vi "Acquisition Message Loop.vi"(8 "error in (no error)":errorcluster, 9 "Data Queue":refnum<queue>, 10 "Data Notifier":refnum<notifier>, 11 "Message Queues":T3) -> (0 "error out":errorcluster)   [LabVIEW 2020, in "Acquisition.lvlib"]
doc: "Message loop for handling messages pertaining to the acquisition of data from the hardware."
uses:
  Acquisition.lvlib
  MESSAGE_QUEUE/All Message Queues.ctl
  MESSAGE_QUEUE/Message Cluster.ctl
  SETTING/data_Queue.ctl
  SETTING/data_Display.ctl
  SETTING/clustOA.ctl
  <vilib>/Analysis/Matrix/Datatypes/RealMatrix.ctl
  HardwareConfiguration.ctl
  CLASS/Image Acquisition Class/Camera.lvclass
  MIRROR/mirror.lvclass
  MIRROR/SIMU_MIRROR/SIMU_MIRROR.lvclass
  D:/USERS/MONTRI/BABYDOL/LABVIEW/EXEMPLE_ARCHITECTURE/acquImageCont_Sav2FITS/MIRROR/mirror.lvclass
  MESSAGE_QUEUE/Message Queue.lvlib
  <vilib>/Analysis/Matrix/NI_Matrix.lvlib
panel:
  out "Cluster 3":cluster{"processedFPS":dbl, "Buffer Number":u32}
  in  "clustPointagFin":T1
  out "File Path Control":path
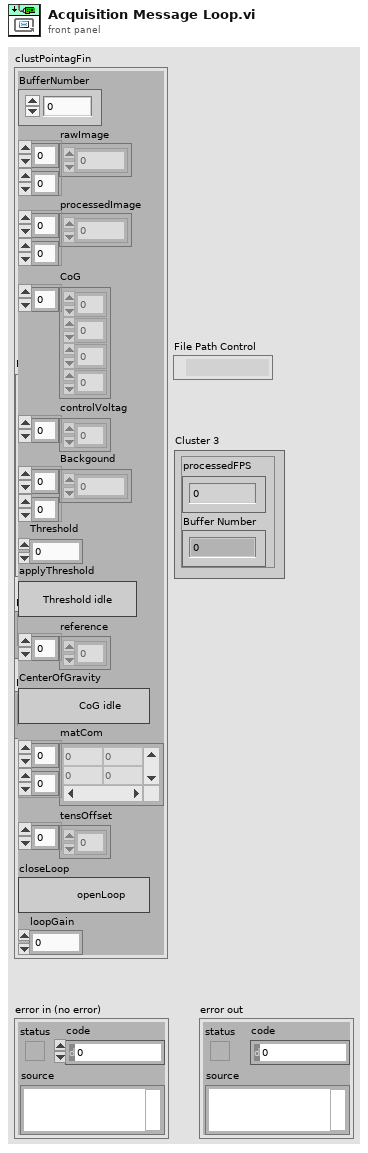
[diagram p1: front panel]
types:
  T1 = typedef "clustOA.ctl" = cluster{"BufferNumber":u32, "rawImage":u16[][], "processedImage":sgl[][], "CoG":dbl[], "controlVoltag":dbl[], "Backgound":sgl[][], "Threshold":dbl, "applyThreshold":bool, "reference":dbl[], "CenterOfGravity":bool, "matCom":T2, "tensOffset":dbl[], "closeLoop":bool, "loopGain":dbl}
  T2 = typedef "NI_Matrix.lvlib/RealMatrix.ctl" = dbl[][]
  T3 = typedef "Message Queue.lvlib/All Message Queues.ctl" = cluster{"UI":refnum<queue>, "Acquisition":refnum<queue>, "Logging":refnum<queue>}
  T4 = typedef "Acquisition.lvlib/HardwareConfiguration.ctl" = cluster{"Camera.lvclass":refnum<class "Camera.lvclass">, "InClusTiming 2":cluster{"Pixelclock":i32, "Exposure":dbl, "ExposureTimeBase":u16, "Framerate":dbl, "TriggerMode":u16}, "ROI":cluster{"PosX":i32, "PosY":i32, "Width":i32, "Height":i32}, "File Path Control":path, "mirror.lvclass":refnum<class "mirror.lvclass">}
  T5 = cluster{"threshold":bool, "thresholdValue (0)":dbl}
  T6 = cluster{"Pixelclock":i32, "Exposure":dbl, "ExposureTimeBase":u16, "Framerate":dbl, "TriggerMode":u16}
  T7 = cluster{"PosX":i32, "PosY":i32, "Width":i32, "Height":i32}
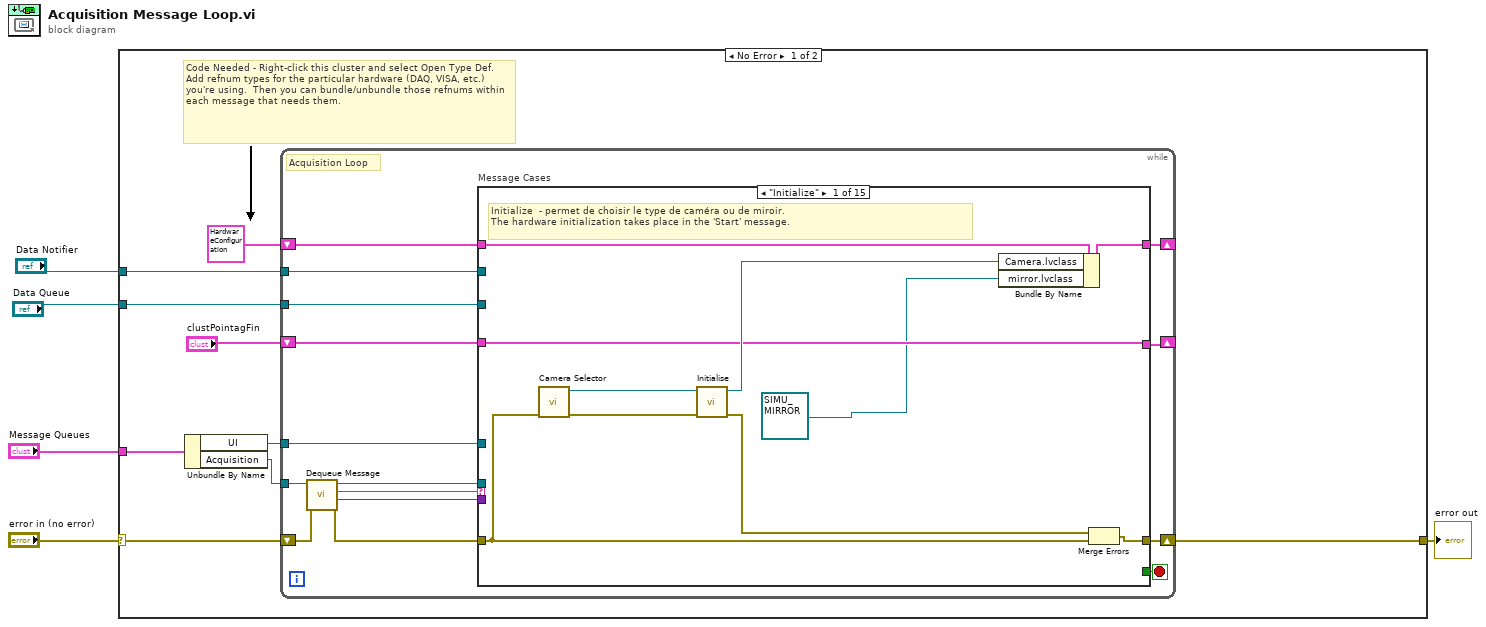
[diagram p0: block diagram]
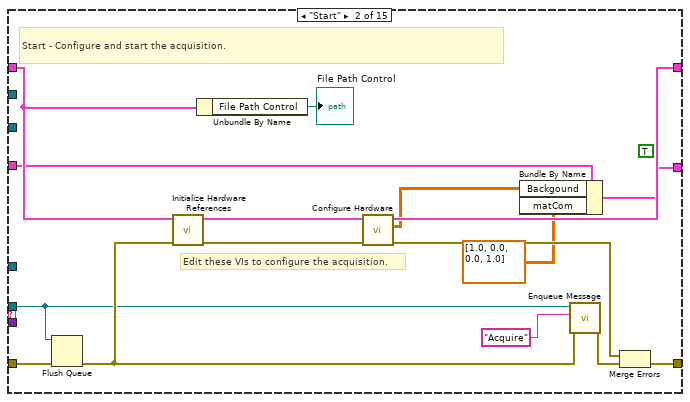
[diagram p2: hidden frame]
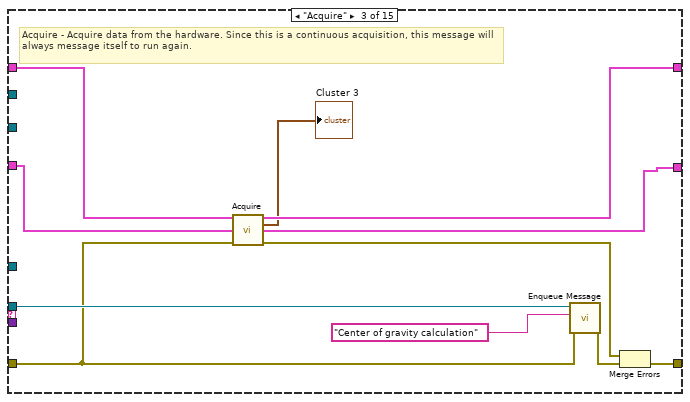
[diagram p3: hidden frame]
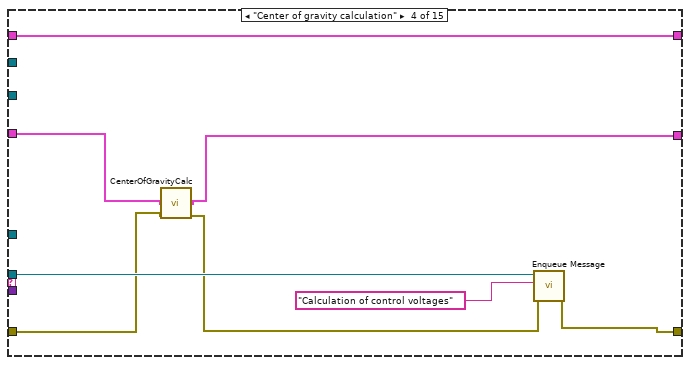
[diagram p4: hidden frame]
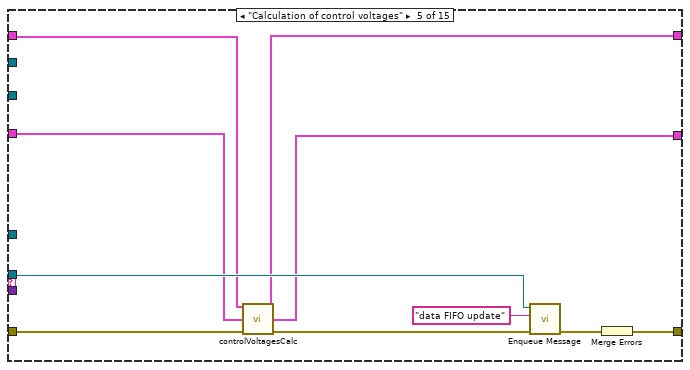
[diagram p5: hidden frame]
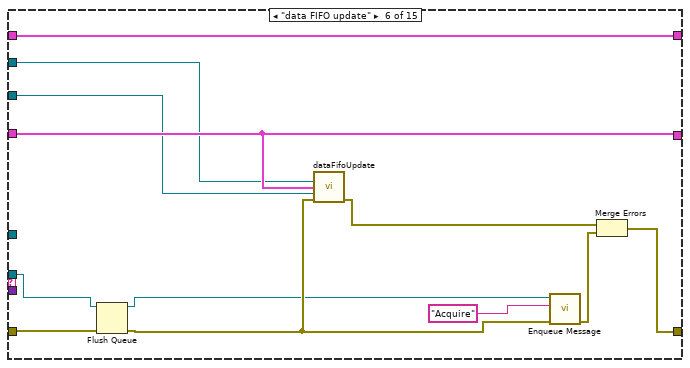
[diagram p6: hidden frame]
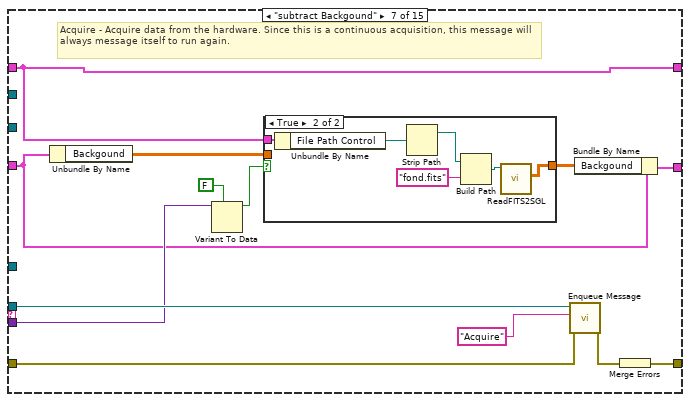
[diagram p7: hidden frame]
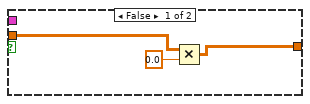
[diagram p8: hidden frame]
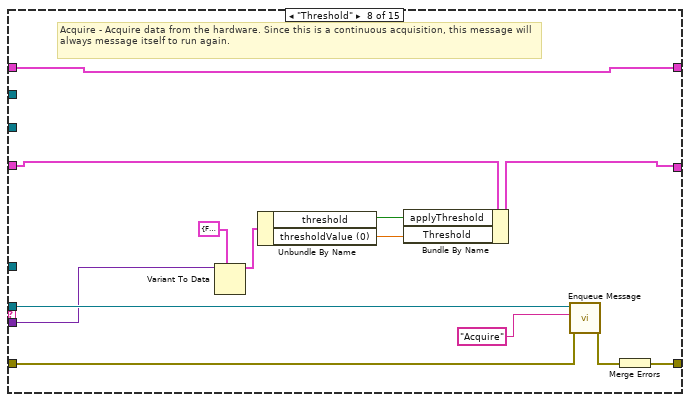
[diagram p9: hidden frame]
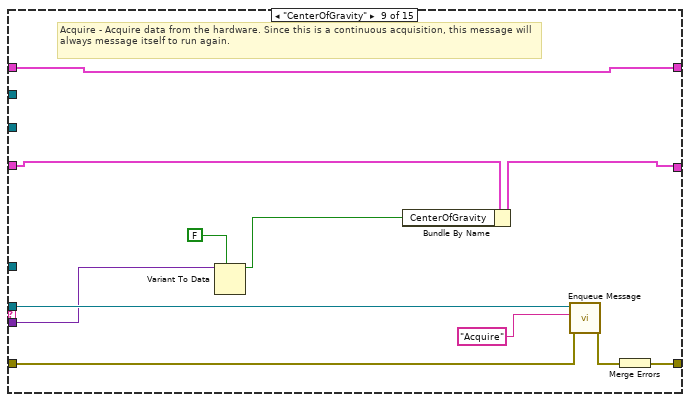
[diagram p10: hidden frame]
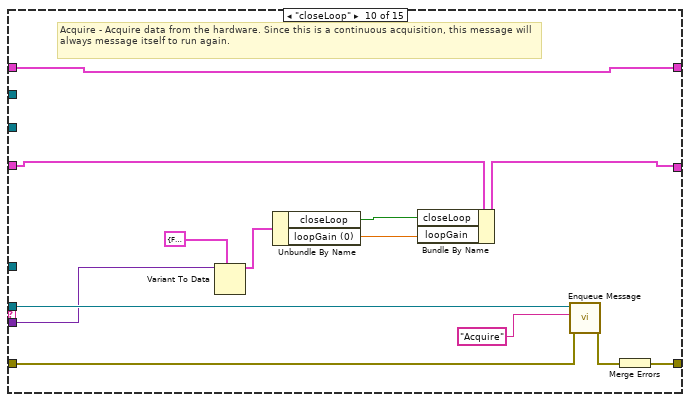
[diagram p11: hidden frame]
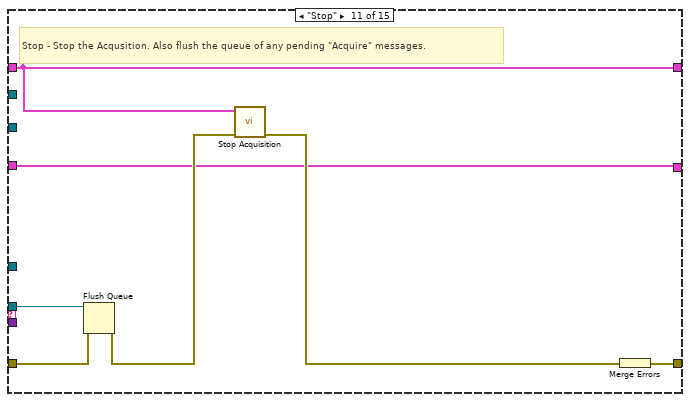
[diagram p12: hidden frame]
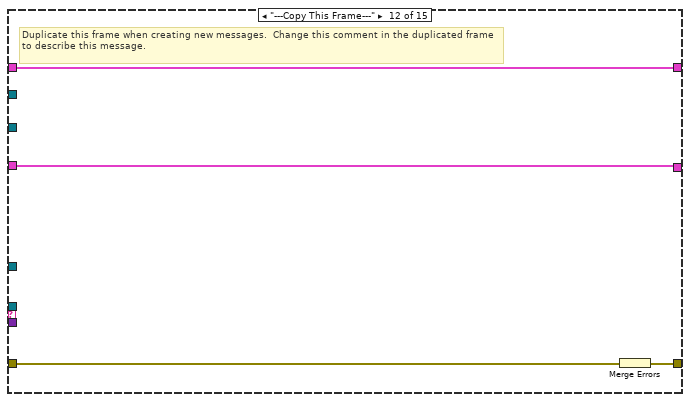
[diagram p13: hidden frame]
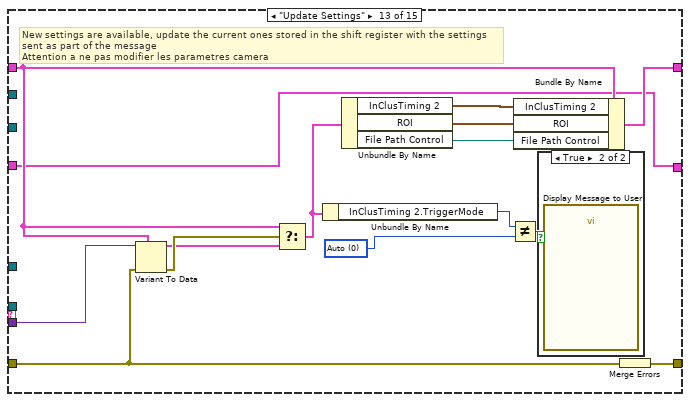
[diagram p14: hidden frame]
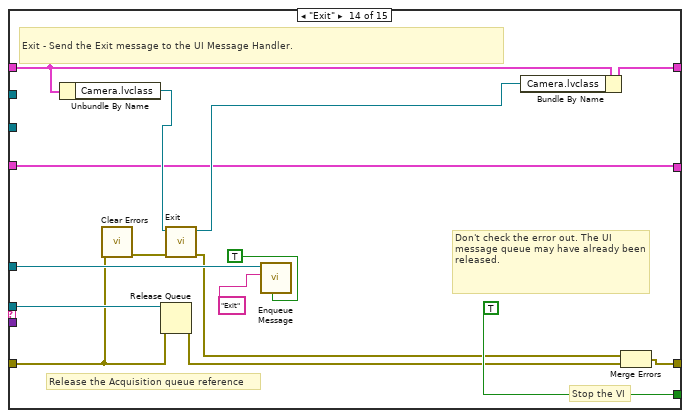
[diagram p16: hidden frame]
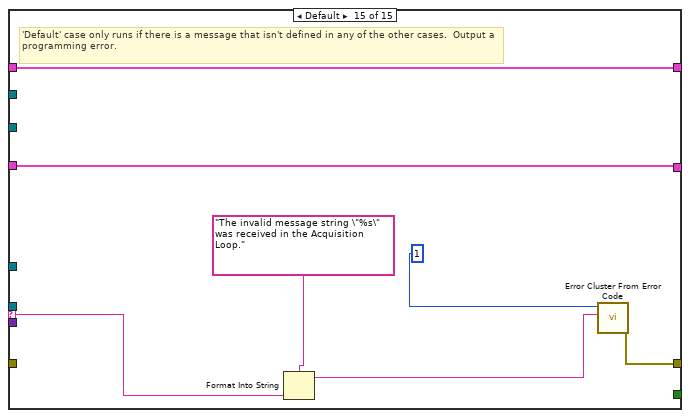
[diagram p17: hidden frame]
diagram:
  n1 = case shown="No Error" "error in (no error)" {
    selector: "error in (no error)" -> [w11 w204]
    tunnel: "Message Queues" -> [w14 _]
    tunnel: [w12 w204] -> w4
    tunnel: "Data Notifier" -> [w9 _]
    tunnel: "Data Queue" -> [w8 _]
    frame No Error {
      # "Code Needed - Right-click this cluster and select Open Type Def.  Add refnum types for the particular hardware (DAQ, VISA, etc.) you're using.  Then you can bundle/unbundle those refnums within each message that needs them."
      n2 = Unbundle By Name(w14) -> ("UI"=w10:refnum<queue>, "Acquisition"=w13:refnum<queue>)
      n3 = while {
        tunnel: w13 -> [w22]
        shift-right: [w28] -> _
        shift-left: T4 {"Camera.lvclass"=refnum, "InClusTiming 2"={"Pixelclock"=0, "Exposure"=0.0, "ExposureTimeBase"=0, "Framerate"=0.0, "TriggerMode"=0}, "ROI"={"PosX"=0, "PosY"=0, "Width"=0, "Height"=0}, "File Path Control"=path "", "mirror.lvclass"=refnum} -> [w29]
        shift-right: [w26] -> w12
        shift-left: w11 -> [w25]
        tunnel: w10 -> [w21]
        tunnel: w9 -> [w20]
        tunnel: w8 -> [w19]
        shift-right: [w15] -> _
        shift-left: "clustPointagFin" -> [w18]
        stop <- w27 stop-if-true
        # "Acquisition Loop"
        n4 = call "Dequeue Message.vi"("error in (no error)"=w25, "Message Queue"=w22) -> ("error out"=w24:errorcluster, "Message Data"=w17:variant, "Message"=w16:string, "dup Message Queue"=w23:refnum<queue>)  [unwired: 6 in]
        n5 = case "Message Cases" shown="\"Initialize\"" w16 {
          selector: w16 -> [_ _ _ _ _ _ _ _ _ _ _ _ _ _ w201]
          tunnel: w23 -> [_ w40 w64 w71 w83 w86 w107 w129 w140 w153 w158 _ _ w190 _]
          tunnel: w24 -> [w32 w42 w63 w68 w80 w88 w106 w128 w139 w152 w161 w166 w177 w189 _]
          tunnel: [w39 w55 w66 w72 w78 w89 w109 w131 w142 w155 w162 w164 w181 w195 w199] -> w26
          tunnel: w29 -> [w38 w48 w59 w74 w77 w95 w104 w126 w137 w150 w157 w165 w176 w186 w203]
          tunnel: [w36 w49 w61 w74 w76 w95 w104 w126 w137 w150 w157 w165 w175 w184 w203] -> w28
          tunnel: [_ _ _ _ _ _ _ _ _ _ _ _ _ TRUE _] -> w27
          tunnel: w17 -> [_ _ _ _ _ _ w103 w125 w136 w149 _ _ w180 _ _]
          tunnel: w21 -> [_ _ _ _ _ _ _ _ _ _ _ _ _ w194 _]
          tunnel: w20 -> [_ _ _ _ _ w92 _ _ _ _ _ _ _ _ _]
          tunnel: w19 -> [_ _ _ _ _ w93 _ _ _ _ _ _ _ _ _]
          tunnel: w18 -> [w31 w46 w58 w70 w82 w94 w100 w124 w135 w148 w156 w163 w167 w182 w197]
          tunnel: [w31 w45 w57 w69 w75 w94 w98 w123 w134 w147 w156 w163 w167 w182 w197] -> w15
          frame "Initialize" {
            # "Initialize  - permet de choisir le type de caméra ou de miroir. \nThe hardware initialization takes place in the 'Start' message."
            n6 = call "Camera Selector.vi"("error in (no error)"=w32) -> ("error out"=w34:errorcluster, "Image Acquisition out"=w33:refnum<class "Camera.lvclass">)  [unwired: 9 in]
            n7 = call-dynamic "Initialise.vi"("error in (no error)"=w34, "Image Acquisition in"=w33) -> ("error out"=w37:errorcluster, "Image Acquisition out"=w35:refnum<class "Camera.lvclass">)  [unwired: 8 in]
            n8 = Bundle By Name(cluster=w38, "Camera.lvclass"=w35, "mirror.lvclass"=refnum<class "SIMU_MIRROR.lvclass"> refnum ("SIMU_MIRROR.lvclass")) -> (w36:T4)
            n9 = Merge Errors(w37, w32) -> (w39:errorcluster)
          }
          frame "Start" {
            (unwired) TRUE ("bUseBuffer0")
            # "Edit these VIs to configure the acquisition."
            # "Start - Configure and start the acquisition."
            n10 = Flush Queue(queue=w40, error in (no error)=w42) -> (error out=w41:errorcluster)  [unwired: 2 out]
            n11 = call "Initialize Hardware References.vi"("error in (no error)"=w41, "Cluster"=w48) -> ("error out"=w53:errorcluster, "Cluster 2"=w50:T4)  [unwired: 8 in]
            n12 = Unbundle By Name(w48) -> ("File Path Control"=→"File Path Control":path)
            n13 = call "Configure Hardware.vi"("error in (no error)"=w53, "Cluster"=w50) -> ("error out"=w52:errorcluster, "initialized array"=w44:sgl[][], "Cluster 2"=w49:T4)  [unwired: 7 in]
            n14 = Bundle By Name(cluster=w46, "Backgound"=w44, "matCom"=T2 [[1.0, 0.0], [0.0, 1.0]]) -> (w45:T1)
            n15 = call "Enqueue Message.vi"("error in (no error)"=w41, "Message"="Acquire", "Message Queue"=w40) -> ("error out"=w54:errorcluster)  [unwired: 7 in, 1 out]
            n16 = Merge Errors(w52, w54) -> (w55:errorcluster)
          }
          frame "Acquire" {
            # "Acquire - Acquire data from the hardware. Since this is a continuous acquisition, this message will always message itself to run again."
            n17 = call "Acquire.vi"("Cluster"=w59, "clustPointagFin"=w58, "error in (no error)"=w63) -> ("Cluster 2"=w61:T4, "clustBufferNumber"=→"Cluster 3":cluster{"processedFPS":dbl, "Buffer Number":u32}, "clustPointagFin"=w57:T1, "error out"=w62:errorcluster)  [unwired: 9 in]
            n18 = call "Enqueue Message.vi"("error in (no error)"=w63, "Message"="Center of gravity calculation", "Message Queue"=w64) -> ("error out"=w65:errorcluster)  [unwired: 7 in, 1 out]
            n19 = Merge Errors(w62, w65) -> (w66:errorcluster)
          }
          frame "Center of gravity calculation" {
            n20 = call "CenterOfGravityCalc.vi"("clustPointagFin"=w70, "error in (no error)"=w68) -> ("clustPointagFin"=w69:T1, "error out"=w67:errorcluster)  [unwired: 12 in]
            n21 = call "Enqueue Message.vi"("error in (no error)"=w67, "Message"="Calculation of control voltages", "Message Queue"=w71) -> ("error out"=w72:errorcluster)  [unwired: 7 in, 1 out]
          }
          frame "Calculation of control voltages" {
            n22 = call "controlVoltagesCalc.vi"("Camera"=w77, "clustPointagFin"=w82, "error in (no error)"=w80) -> ("output cluster"=w76:T4, "clustPointagFin"=w75:T1, "error out"=w81:errorcluster)  [unwired: 10 in]
            n23 = call "Enqueue Message.vi"("error in (no error)"=w81, "Message"="data FIFO update", "Message Queue"=w83) -> ("error out"=w79:errorcluster)  [unwired: 7 in, 1 out]
            n24 = Merge Errors(w79) -> (w78:errorcluster)
          }
          frame "data FIFO update" {
            n25 = Flush Queue(queue=w86, error in (no error)=w88) -> (queue out=w85:refnum<queue>, error out=w87:errorcluster)  [unwired: 1 out]
            n26 = call "dataFifoUpdate.vi"("Data Notifier"=w92, "clustPointagFin"=w94, "Data Queue"=w93, "error in (no error)"=w87) -> ("error out"=w91:errorcluster)  [unwired: 11 in]
            n27 = call "Enqueue Message.vi"("error in (no error)"=w87, "Message"="Acquire", "Message Queue"=w85) -> ("error out"=w90:errorcluster)  [unwired: 7 in, 1 out]
            n28 = Merge Errors(w91, w90) -> (w89:errorcluster)
          }
          frame "subtract Backgound" {
            # "Acquire - Acquire data from the hardware. Since this is a continuous acquisition, this message will always message itself to run again."
            n29 = Unbundle By Name(w100) -> ("Backgound"=w99:sgl[][])
            n30 = Variant To Data(type=FALSE, Variant=w103) -> (data=w101:bool)  [unwired: 1 in, 1 out]
            n31 = case shown="True" w101 {
              tunnel: w104 -> [_ w118]
              tunnel: [w111 w117] -> w97
              tunnel: w99 -> [w110 _]
              frame False {
                n32 = Multiply(x=w110, y=sgl 0.0) -> (x*y=w111:sgl[][])
              }
              frame True {
                n33 = Unbundle By Name(w118) -> ("File Path Control"=w114:path)
                n34 = Strip Path(path=w114) -> (stripped path=w113:path)  [unwired: 1 out]
                n35 = Build Path(base path=w113, name or relative path="fond.fits") -> (appended path=w115:path)
                n36 = call "ReadFITS2SGL.vi"("Path"=w115) -> ("Tableau2DSGL"=w117:sgl[][])  [unwired: 7 in, 3 out]
              }
            }
            n37 = call "Enqueue Message.vi"("error in (no error)"=w106, "Message"="Acquire", "Message Queue"=w107) -> ("error out"=w108:errorcluster)  [unwired: 7 in, 1 out]
            n38 = Bundle By Name(cluster=w100, "Backgound"=w97) -> (w98:T1)
            n39 = Merge Errors(w108) -> (w109:errorcluster)
          }
          frame "Threshold" {
            # "Acquire - Acquire data from the hardware. Since this is a continuous acquisition, this message will always message itself to run again."
            n40 = Variant To Data(type=T5 {"threshold"=FALSE, "thresholdValue (0)"=0.0}, Variant=w125) -> (data=w121:T5)  [unwired: 1 in, 1 out]
            n41 = Unbundle By Name(w121) -> ("threshold"=w119:bool, "thresholdValue (0)"=w120:dbl)
            n42 = Bundle By Name(cluster=w124, "applyThreshold"=w119, "Threshold"=w120) -> (w123:T1)
            n43 = call "Enqueue Message.vi"("error in (no error)"=w128, "Message"="Acquire", "Message Queue"=w129) -> ("error out"=w130:errorcluster)  [unwired: 7 in, 1 out]
            n44 = Merge Errors(w130) -> (w131:errorcluster)
          }
          frame "CenterOfGravity" {
            # "Acquire - Acquire data from the hardware. Since this is a continuous acquisition, this message will always message itself to run again."
            n45 = Variant To Data(type=FALSE, Variant=w136) -> (data=w132:bool)  [unwired: 1 in, 1 out]
            n46 = Bundle By Name(cluster=w135, "CenterOfGravity"=w132) -> (w134:T1)
            n47 = call "Enqueue Message.vi"("error in (no error)"=w139, "Message"="Acquire", "Message Queue"=w140) -> ("error out"=w141:errorcluster)  [unwired: 7 in, 1 out]
            n48 = Merge Errors(w141) -> (w142:errorcluster)
          }
          frame "closeLoop" {
            # "Acquire - Acquire data from the hardware. Since this is a continuous acquisition, this message will always message itself to run again."
            n49 = Variant To Data(type=cluster{"closeLoop":bool, "loopGain (0)":dbl} {"closeLoop"=FALSE, "loopGain (0)"=0.0}, Variant=w149) -> (data=w146:cluster{"closeLoop":bool, "loopGain (0)":dbl})  [unwired: 1 in, 1 out]
            n50 = Unbundle By Name(w146) -> ("closeLoop"=w144:bool, "loopGain (0)"=w145:dbl)
            n51 = Bundle By Name(cluster=w148, "closeLoop"=w144, "loopGain"=w145) -> (w147:T1)
            n52 = call "Enqueue Message.vi"("error in (no error)"=w152, "Message"="Acquire", "Message Queue"=w153) -> ("error out"=w154:errorcluster)  [unwired: 7 in, 1 out]
            n53 = Merge Errors(w154) -> (w155:errorcluster)
          }
          frame "Stop" {
            # "Stop - Stop the Acqusition. Also flush the queue of any pending \"Acquire\" messages."
            n54 = Flush Queue(queue=w158, error in (no error)=w161) -> (error out=w159:errorcluster)  [unwired: 2 out]
            n55 = call "Stop Acquisition.vi"("error in (no error)"=w159, "Cluster"=w157) -> ("error out"=w160:errorcluster)  [unwired: 8 in, 1 out]
            n56 = Merge Errors(w160) -> (w162:errorcluster)
          }
          frame "---Copy This Frame---" {
            # "Duplicate this frame when creating new messages.  Change this comment in the duplicated frame to describe this message."
            n57 = Merge Errors(w166) -> (w164:errorcluster)
          }
          frame "Update Settings" {
            w169 = u16 0 items=["Auto", "Software", "External sequence start ", "External exposure control"] ("TriggerMode")
            # "New settings are available, update the current ones stored in the shift register with the settings sent as part of the message\nAttention a ne pas modifier les parametres camera"
            n58 = Variant To Data(error in=w177, type=w176, Variant=w180) -> (data=w178:T4, error out=w179:errorcluster)
            n59 = Select(t=w176, s=w179, f=w178) -> (s? t:f=w171:T4)
            n60 = Unbundle By Name(w171) -> ("InClusTiming 2.TriggerMode"=w170:u16)
            n61 = Unbundle By Name(w171) -> ("InClusTiming 2"=w174:T6, "ROI"=w173:T7, "File Path Control"=w172:path)
            n62 = Not Equal?(x=w170, y=w169) -> (x != y?=w168:bool)
            n63 = Bundle By Name(cluster=w176, "InClusTiming 2"=w174, "ROI"=w173, "File Path Control"=w172) -> (w175:T4)
            n64 = case shown="True" w168 {
              frame False {
              }
              frame True {
                n65 = call "Display Message to User"() -> ()  [unwired: 10 in, 2 out]
              }
            }
            n66 = Merge Errors(w177) -> (w181:errorcluster)
          }
          frame "Exit" {
            # "Don't check the error out. The UI message queue may have already been released."
            # "Release the Acquisition queue reference"
            # "Stop the VI"
            # "Exit - Send the Exit message to the UI Message Handler."
            n67 = Unbundle By Name(w186) -> ("Camera.lvclass"=w185:refnum<class "Camera.lvclass">)
            n68 = call <vilib>:"Clear Errors.vi"("error in (no error)"=w189) -> ("error out"=w187:errorcluster)  [unwired: 5 in, 1 out]
            n69 = Release Queue(queue=w190, error in (no error)=w189) -> (error out=w191:errorcluster)  [unwired: 1 in, 2 out]
            n70 = call-dynamic "Exit.vi"("error in (no error)"=w187, "Image Acquisition in"=w185) -> ("error out"=w188:errorcluster, "Image Acquisition out"=w183:refnum<class "Camera.lvclass">)  [unwired: 8 in]
            n71 = call "Enqueue Message.vi"("Priority Message? (F)"=TRUE, "Message"="Exit", "Message Queue"=w194) -> ()  [unwired: 7 in, 2 out]
            n72 = Bundle By Name(cluster=w186, "Camera.lvclass"=w183) -> (w184:T4)
            n73 = Merge Errors(w188, w191) -> (w195:errorcluster)
          }
          frame Default {
            # "'Default' case only runs if there is a message that isn't defined in any of the other cases.  Output a programming error."
            n74 = Format Into String(format string="The invalid message string \"%s\" was received in the Acquisition Loop." ("Invalid Acquisition Message"), w201) -> (resulting string=w198:string)  [unwired: 2 in, 1 out]
            n75 = call <vilib>:"Error Cluster From Error Code.vi"("error message (\"\")"=w198, "error code (0)"=1) -> ("error out"=w199:errorcluster)  [unwired: 7 in]
          }
        }
      }
    }
    frame Error {
    }
  }
  "error out" <- w4
